vi "test-PID-setUpBeforeClass.vi"(8 "error in (no error)":errorcluster) -> (0 "error out":errorcluster)   [LabVIEW 2019]
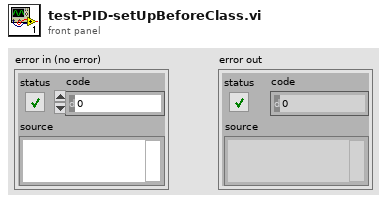
[diagram p1: front panel]
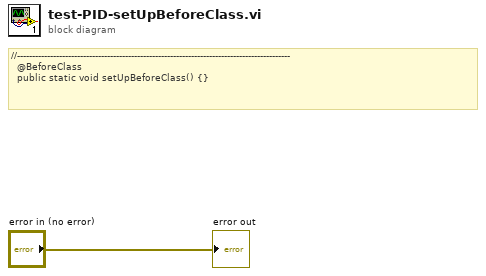
[diagram p0: block diagram]
diagram:
  # "//-------------------------------------------------------------------------------------------\n  @BeforeClass\n  public static void setUpBeforeClass() {}"
  "error out" <- "error in (no error)"
